vi "Write VI Refnum-Main.vi"(8 "error in (no error)":errorcluster, 10 "VI Refnum-Main":refnum<vi>, 11 "FE FF Frame in":refnum<class "FE FF Frame.lvclass">) -> (0 "error out":errorcluster, 3 "FE FF Frame out":refnum<class "FE FF Frame.lvclass">)   [LabVIEW 2023, in "Data Analysis.lvlib" / "FE FF Frame.lvlib" / "FE FF Frame.lvclass"]
uses:
  FE FF Frame.lvclass
  FE FF Frame.lvclass/FE FF Frame.ctl
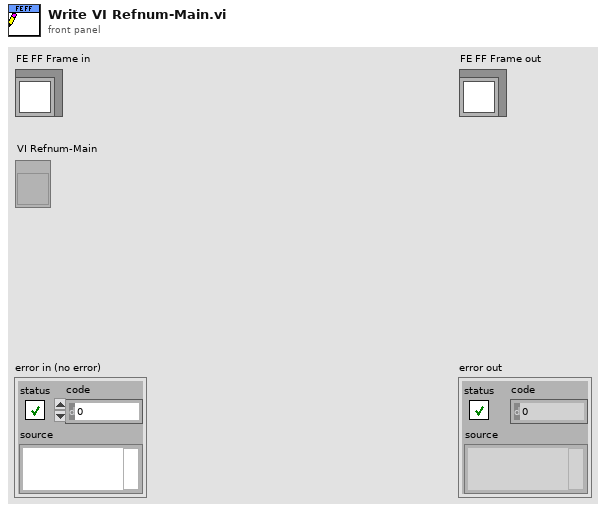
[diagram p1: front panel]
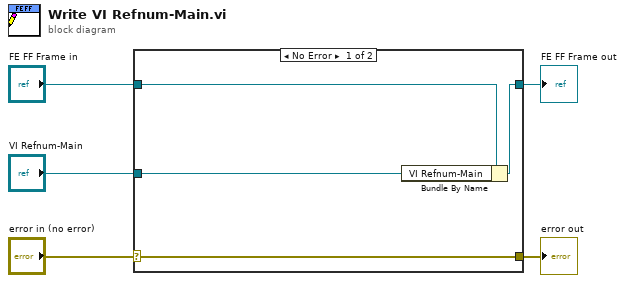
[diagram p0: block diagram]
diagram:
  n1 = case shown="No Error" "error in (no error)" {
    selector: "error in (no error)" -> [w9 w10]
    tunnel: [w9 w10] -> w4
    tunnel: [w7 w11] -> w2
    tunnel: "FE FF Frame in" -> [w8 w11]
    tunnel: "VI Refnum-Main" -> [w6 _]
    frame No Error {
      n2 = Bundle By Name(cluster=w8, "VI Refnum-Main"=w6) -> (w7:refnum<class "FE FF Frame.lvclass">)
    }
    frame Error {
    }
  }
  "error out" <- w4
  "FE FF Frame out" <- w2
